vi "Min Read Array.vi"(8 "error in":errorcluster, 11 "Min Power Limit in":refnum<class "Power Limit.lvclass">) -> (0 "error out":errorcluster, 1 "Changed or First Call?":bool, 2 "Current Min Limit":dbl[](array[numeric]), 3 "Min Power Limit out":refnum<class "Power Limit.lvclass">)   [LabVIEW 2023, in "Power Limit.lvclass"]
uses:
  Power Limit.lvclass
  Parents/Limit/Limit.lvclass
  Power Limit.lvclass/Power Limit.ctl
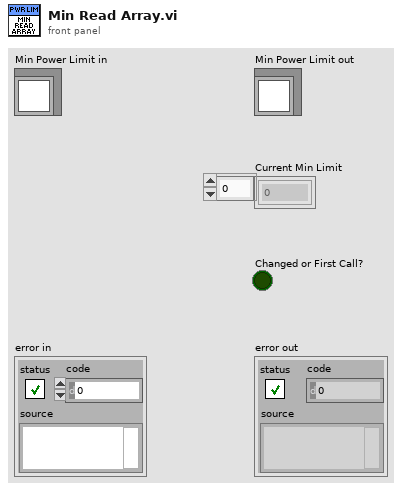
[diagram p1: front panel]
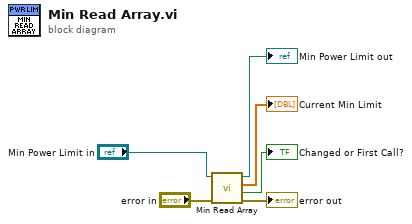
[diagram p0: block diagram]
diagram:
  n1 = call-parent "Min Read Array.vi"("error in"="error in", "Min Limit in"="Min Power Limit in") -> ("error out"=→"error out":errorcluster, "Changed or First Call?"=→"Changed or First Call?":bool, "Current Min Limit"=→"Current Min Limit":dbl[], "Min Limit out"=→"Min Power Limit out":refnum<class "Power Limit.lvclass">)  [unwired: 6 in]
